vi "SUB-BLE SCAN.vi"(5 "Port-set 1":refnum<visa-resource-name>="COM8" caption="COM port") -> (0 "Device Name":string, 1 "Connection Status":T1={"MAC Address"="D9:2F:10:92:34:F2", "cnx handle"=0, "cnx flags"=5, "Address Type"=1, "Connection Interval (ms)"=15, "Timeout(ms)"=1000, "Latency"=0, "bonding handle"=255} {"Address Type" items=["Public", "Random"]}, 2 "Connected":bool)   [LabVIEW 2015]
doc: "Use this template to create an application that executes repeatedly until you click the Stop button. This template polls the state of the Stop button and does not use events. Use the Top-Level Application template (not available in the Base package) to create a single-loop application with event handling."
uses:
  Lib_Bled112 toolkit/type_def/connection_status_bundle.ctl
  Lib_Bled112 toolkit/type_def/address_type.ctl
panel:
  out "Handle table":string[][](array[string])
  out "Address Type":enum16{"Public", "Random"}(ring)=enum."Random"
  out "MAC Address":string="D9:2F:10:92:34:F2"
  in  "최소":bool
  in  "연결":bool
  in  "새로 검색":bool
  out "검색시작":bool caption="검색 시작"
  out "Complete":bool
  in  "Device List":i32(listbox)=2
  out "Scanning":bool
  # "Device Select"
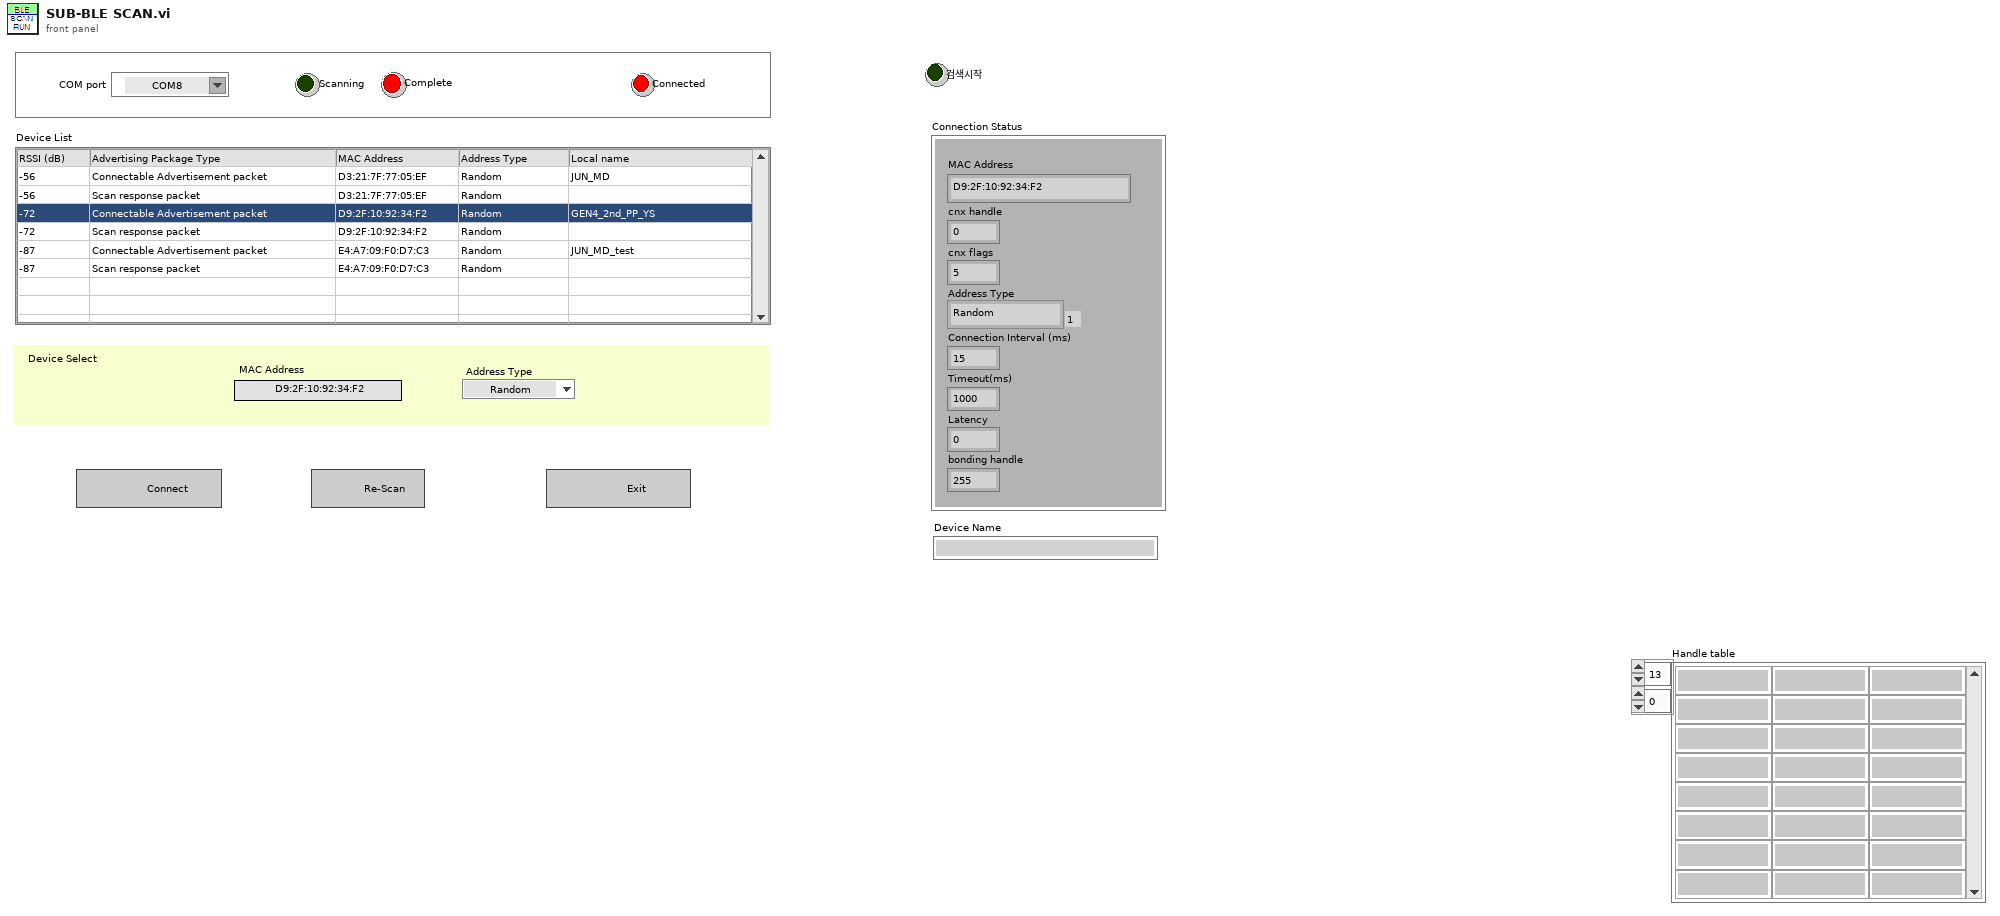
[diagram p1: front panel]
types:
  T1 = typedef "connection_status_bundle.ctl" = cluster{"MAC Address":string, "cnx handle":u8, "cnx flags":u8, "Address Type":T2, "Connection Interval (ms)":u16, "Timeout(ms)":u16, "Latency":u16, "bonding handle":u8}
  T2 = typedef "address_type.ctl" = u8
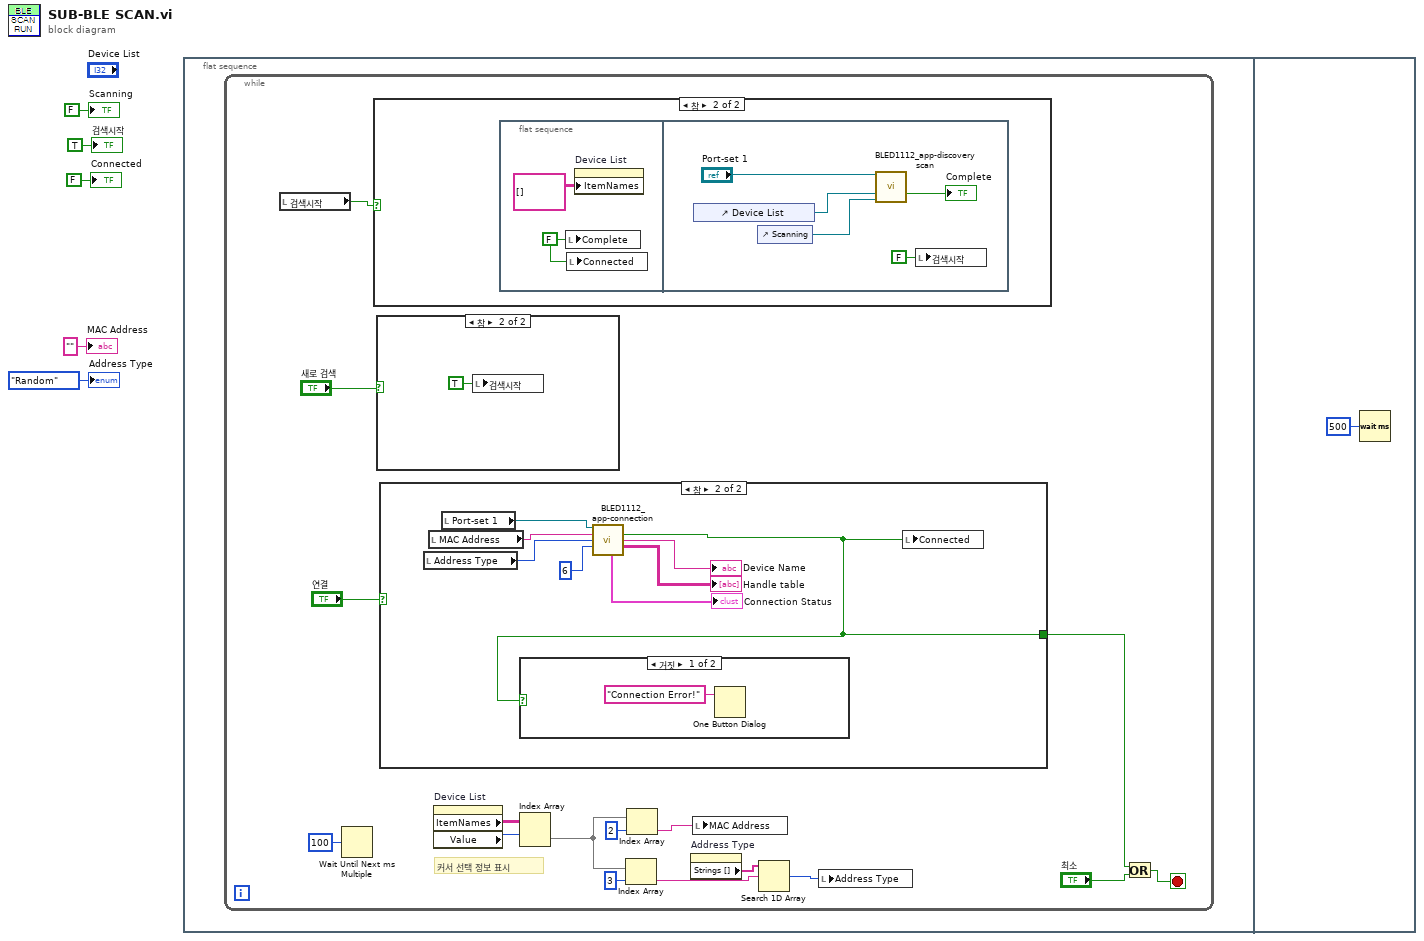
[diagram p0: block diagram]
diagram:
  n1 = flat-sequence {
    frame #0 {
      n2 = while {
        stop <- w6 stop-if-true
        # "커서 선택 정보 표시"
        n3 = local read "검색시작"() -> (w21:bool)
        n4 = Wait Until Next ms Multiple(millisecond multiple=u32 100 ("ms 배수")) -> ()  [unwired: 1 out]
        n5 = case shown="참" w21 {
          frame False {
          }
          frame True {
            n6 = flat-sequence {
              frame #0 {
                w32 = FALSE ("검색 완료")
                n7 = local write "Complete"(w32) -> ()
                n8 = local write "Connected"(w32) -> ()
                n9 = property on="Device List" class="MCListbox (엄격한)"("ItemNames"=string[][] [] ("아이템 이름")) -> ()  [unwired: 2 in, 2 out]
              }
              frame #1 {
                n10 = control-ref of="Device List"() -> (w35:refnum<vi>)
                n11 = control-ref of="Scanning"() -> (w36:refnum<vi>)
                n12 = call "BLED1112_app-discovery scan.vi"("COM in"="Port-set 1", "Device List"=w35, "LED ref"=w36) -> ("Scan success?"=→"Complete":bool)  [unwired: 8 in, 4 out]
                n13 = local write "검색시작"(FALSE ("검색시작")) -> ()
              }
            }
          }
        }
        n14 = case shown="참" "새로 검색" {
          frame False {
          }
          frame True {
            n15 = local write "검색시작"(TRUE ("검색시작")) -> ()
          }
        }
        n16 = case shown="참" "연결" {
          tunnel: [_ w22] -> w7
          frame False {
          }
          frame True {
            n17 = local read "Address Type"() -> (w23:enum16{"Public", "Random"})
            n18 = local read "MAC Address"() -> (w24:string)
            n19 = local read "Port-set 1"() -> (w25:refnum<visa-resource-name>)
            n20 = call "BLED1112_app-connection.vi"("COM Bluegiga in"=w25, "MAC Address"=w24, "Address Type"=w23, "Conn Try no"=6) -> ("Connection Ok"=w22:bool, "Device Name"=→"Device Name":string, "Handle table"=→"Handle table":string[][], "Connection Status"=→"Connection Status":T1)  [unwired: 6 in, 2 out]
            n21 = case shown="거짓" w22 {
              frame False {
                n22 = One Button Dialog(message="Connection Error!" ("메시지")) -> ()  [unwired: 1 in, 1 out]
              }
              frame True {
              }
            }
            n23 = local write "Connected"(w22) -> ()
          }
        }
        n24 = property on="Device List" class="MCListbox (엄격한)"() -> ("ItemNames"=w20:string[][], "Value"=w19:i32)  [unwired: 2 in, 2 out]
        n25 = Index Array(array=w20, index (row)=w19) -> (element=w15:string[])  [unwired: 1 in]
        n26 = Index Array(array=w15, index=3 ("인덱스")) -> (element=w14:string)
        n27 = Index Array(array=w15, index=2 ("인덱스")) -> (element=w17:string)
        n28 = property on="Address Type" class="Enum (엄격한)"() -> ("Strings []"=w12:string[])  [unwired: 2 in, 2 out]
        n29 = local write "MAC Address"(w17) -> ()
        n30 = Search 1D Array(1D array=w12, element=w14) -> (index of element=w13:i32)  [unwired: 1 in]
        n31 = local write "Address Type"(w13) -> ()
        n32 = Or(x=w7, y="최소") -> (x .or. y?=w6:bool)
      }
    }
    frame #1 {
      n33 = Wait (ms)(milliseconds to wait=u32 500 ("대기 시간(ms)")) -> ()  [unwired: 1 out]
    }
  }
  "Scanning" <- FALSE ("Scanning")
  "검색시작" <- TRUE ("검색시작")
  "Connected" <- FALSE ("Connected")
  "MAC Address" <- "" ("MAC Address")
  "Address Type" <- enum16{"Public", "Random"}."Random" ("Address Type")
